vi "Navigation_Alex_auto.vi"() -> ()   [LabVIEW 2015]
uses:
  <vilib>/myRIO/Instrument Drivers/Utilities/Utilities.lvlib
  <vilib>/rvi/interface/nirviReadWriteControl/nirviReadWriteControl.xnode
  NiFpgaLv.dll
  <vilib>/Utility/error.llb/Error Cluster From Error Code.vi
  <vilib>/rvi/interface/Simulation/niFpgaSimulationCallBeginRW.vi
  <vilib>/rvi/errors/niLvFpgaAdjustHostInterfaceError.vi
  <vilib>/rvi/interface/nirviOpenFPGA/nirviOpenFPGA.xnode
  FPGA Bitfiles/NavigationProjec_FPGATarget2_FPGAMainNavigati_PWPHW8gwDxI.lvbitx
  <vilib>/FPGAPlugInAG/myRIO-1900/niLvFpga_Open_myRIO-1900.vi
  <vilib>/rvi/interface/common/dynamic/niFpgaDynamicAddResources.vi
  <vilib>/myRIO/Instrument Drivers/Onboard IO/PWM/typedefs/PWM Configuration.ctl
  <vilib>/myRIO/Instrument Drivers/Onboard IO/PWM/PWM.lvlib
  <vilib>/myRIO/Common/Instrument Driver Framework/myRIO v1.0/PWM/typedefs/PWM Channels Enum.ctl
  <vilib>/myRIO/Common/Instrument Driver Framework/Utilities/typedefs/Generic FPGA Reference.ctl
  <vilib>/myRIO/Common/Instrument Driver Framework/Utilities/typedefs/myRIO v1.0 Reference.ctl
  <vilib>/myRIO/Common/Instrument Driver Framework/Utilities/typedefs/Hardware Version Enum.ctl
  <vilib>/myRIO/Common/Instrument Driver Framework/Utilities/typedefs/myRIO Generic Hardware Reference.ctl
  <vilib>/myRIO/Instrument Drivers/Onboard IO/PWM/typedefs/PWM Reference.ctl
  <vilib>/myRIO/Instrument Drivers/Onboard IO/PWM/vis/myRIO PWM Open.xnode
  <vilib>/myRIO/Common/Instrument Driver Framework/myRIO v1.0/PWM/vis/myRIO v1.1 Open PWM.vi
  <vilib>/userdefined/High Color/nirio_resource_hc.ctl
panel:
  in  "Right PWM":dbl
  in  "Left PWM":dbl
  in  "Goal X":dbl
  out "Right Setpoint":dbl
  out "Current Angle":dbl
  out "Current Y":dbl
  out "Current X":dbl
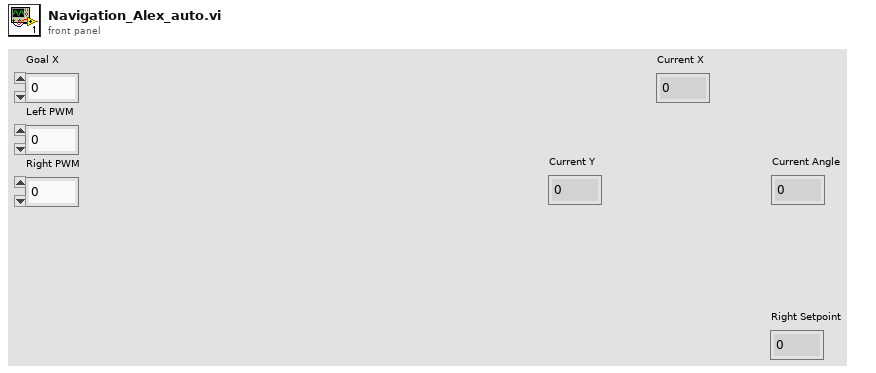
[diagram p1: front panel]
types:
  T1 = typedef "nirio_resource_hc.ctl" = tag
  T2 = typedef "Hardware Version Enum.ctl" = enum16{"Unknown", "myRIO-1900", "myRIO-1950", "roboRIO"}
  T3 = typedef "PWM.lvlib/PWM Reference.ctl" = cluster{"myRIO Reference":T4, "PWM Channels Enum":T7, "PWM Configuration":T8}
  T4 = typedef "myRIO Generic Hardware Reference.ctl" = cluster{"myRIO Model":T2, "myRIO Hardware Reference":T5}
  T5 = typedef "myRIO v1.0 Reference.ctl" = cluster{"Generic FPGA Reference":T6, "Allow multiple opens":bool}
  T6 = typedef "Generic FPGA Reference.ctl" = refnum<k20>
  T7 = typedef "PWM Channels Enum.ctl" = enum16{"Not Connected", "C/PWM0", "C/PWM1", "A/PWM0", "A/PWM1", "A/PWM2", "B/PWM0", "B/PWM1", "B/PWM2", "PWM/PWM0", "PWM/PWM1", "PWM/PWM2", "PWM/PWM3", "PWM/PWM4", "PWM/PWM5", "PWM/PWM6", "PWM/PWM7", "PWM/PWM8", "PWM/PWM9"}
  T8 = typedef "PWM.lvlib/PWM Configuration.ctl" = cluster{"Frequency":dbl, "Duty Cycle":dbl}
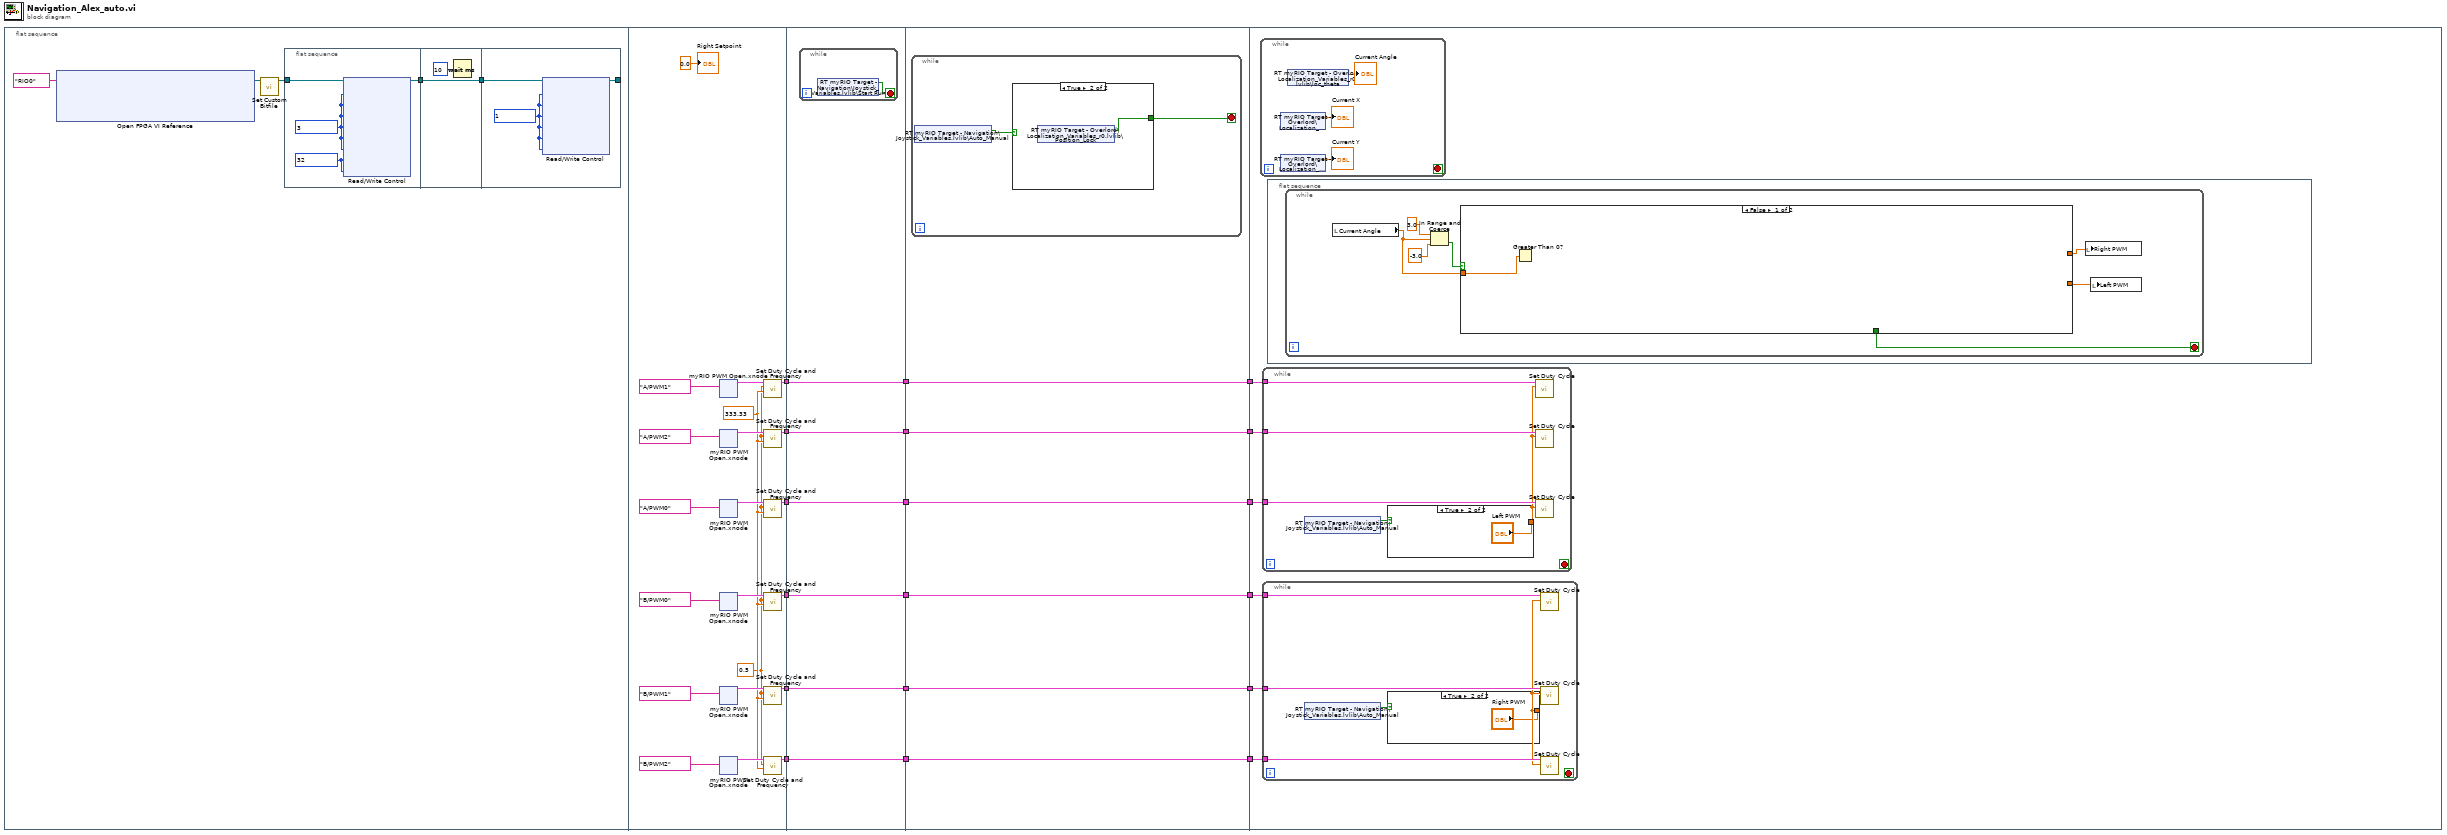
[diagram p0: block diagram]
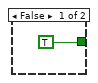
[diagram p2: hidden frame]
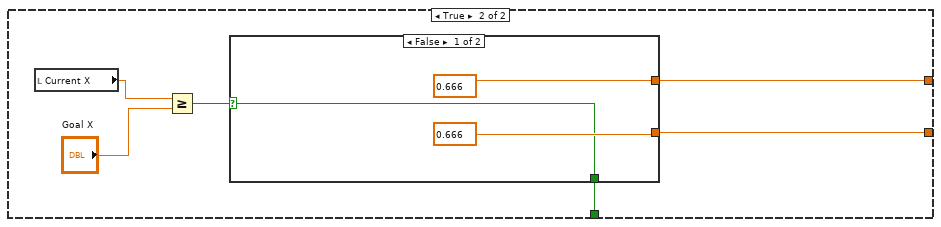
[diagram p3: hidden frame]
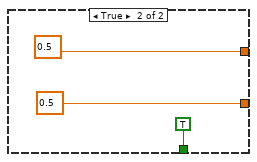
[diagram p4: hidden frame]
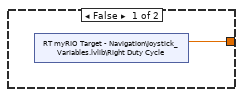
[diagram p5: hidden frame]
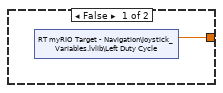
[diagram p6: hidden frame]
diagram:
  n1 = flat-sequence {
    tunnel: [w39] -> w18
    tunnel: [w38] -> w17
    tunnel: [w37] -> w16
    tunnel: [w36] -> w15
    tunnel: [w35] -> w14
    tunnel: [w34] -> w13
    tunnel: w18 -> [w155]
    tunnel: w17 -> [w154]
    tunnel: w16 -> [w153]
    tunnel: w15 -> [w152]
    tunnel: w14 -> [w151]
    tunnel: w13 -> [w150]
    tunnel: [w155] -> w12
    tunnel: [w154] -> w11
    tunnel: [w153] -> w10
    tunnel: [w152] -> w9
    tunnel: [w151] -> w8
    tunnel: [w150] -> w7
    tunnel: w12 -> [w162]
    tunnel: w11 -> [w161]
    tunnel: w10 -> [w160]
    tunnel: w9 -> [w159]
    tunnel: w8 -> [w158]
    tunnel: w7 -> [w157]
    tunnel: [w162] -> w6
    tunnel: [w161] -> w5
    tunnel: [w160] -> w4
    tunnel: [w159] -> w3
    tunnel: [w158] -> w2
    tunnel: [w157] -> w1
    tunnel: w1 -> [w169]
    tunnel: w2 -> [w168]
    tunnel: w3 -> [w167]
    tunnel: w4 -> [w170]
    tunnel: w5 -> [w171]
    tunnel: w6 -> [w172]
    frame #0 {
      n2 = xnode "Open FPGA VI Reference"("resource name"=tag "RIO0") -> ("FPGA VI Reference Out"=w20:refnum<k20>)  [unwired: 1 in, 1 out]
      n3 = call <vilib>:"Set Custom Bitfile.vi"("Custom FPGA Reference In"=w20) -> ("Custom FPGA Reference Out"=w21:refnum<k20>)  [unwired: 9 in, 1 out]
      n4 = flat-sequence {
        tunnel: w21 -> [w26]
        tunnel: [w24] -> w23
        tunnel: w23 -> [w28]
        tunnel: [w28] -> w22
        tunnel: w22 -> [w31]
        tunnel: [w30] -> _
        frame #0 {
          w25 = u8 32 ("SYS.SELECTA")
          w27 = u8 3 ("ENC.B_c.CNFG")
          n5 = xnode "Read/Write Control"("FPGA VI Reference In"=w26, "ENC.A_a.CNFG"=w27, "ENC.A_b.CNFG"=w27, "ENC.A_c.CNFG"=w27, "ENC.B_a.CNFG"=w27, "ENC.B_b.CNFG"=w27, "ENC.B_c.CNFG"=w27, "SYS.SELECTA"=w25, "SYS.SELECTB"=w25) -> ("FPGA VI Reference Out"=w24:refnum<k20>)  [unwired: 1 in, 1 out]
        }
        frame #1 {
          n6 = Wait (ms)(milliseconds to wait=u32 10) -> ()  [unwired: 1 out]
        }
        frame #2 {
          w32 = u8 1 ("ENC.B_c.CNFG")
          n7 = xnode "Read/Write Control"("FPGA VI Reference In"=w31, "ENC.A_a.CNFG"=w32, "ENC.A_b.CNFG"=w32, "ENC.A_c.CNFG"=w32, "ENC.B_a.CNFG"=w32, "ENC.B_b.CNFG"=w32, "ENC.B_c.CNFG"=w32) -> ("FPGA VI Reference Out"=w30:refnum<k20>)  [unwired: 1 in, 1 out]
        }
      }
    }
    frame #1 {
      w40 = 0.5
      w41 = 333.33
      n8 = xnode "myRIO PWM Open.xnode"("Channel Name"=tag "A/PWM1") -> ("PWM Ref Out"=w46:T3)  [unwired: 2 in, 1 out]
      n9 = xnode "myRIO PWM Open.xnode"("Channel Name"=tag "A/PWM2") -> ("PWM Ref Out"=w45:T3)  [unwired: 2 in, 1 out]
      n10 = xnode "myRIO PWM Open.xnode"("Channel Name"=tag "A/PWM0") -> ("PWM Ref Out"=w47:T3)  [unwired: 2 in, 1 out]
      n11 = xnode "myRIO PWM Open.xnode"("Channel Name"=tag "B/PWM0") -> ("PWM Ref Out"=w44:T3)  [unwired: 2 in, 1 out]
      n12 = xnode "myRIO PWM Open.xnode"("Channel Name"=tag "B/PWM1") -> ("PWM Ref Out"=w43:T3)  [unwired: 2 in, 1 out]
      n13 = xnode "myRIO PWM Open.xnode"("Channel Name"=tag "B/PWM2") -> ("PWM Ref Out"=w42:T3)  [unwired: 2 in, 1 out]
      n14 = call <vilib>:"Set Duty Cycle and Frequency.vi"("Frequency [Hz]"=w41, "Duty Cycle"=w40, "PWM Ref In"=w46) -> ("PWM Ref Out"=w38:T3)  [unwired: 6 in, 1 out]
      n15 = call <vilib>:"Set Duty Cycle and Frequency.vi"("Frequency [Hz]"=w41, "Duty Cycle"=w40, "PWM Ref In"=w45) -> ("PWM Ref Out"=w37:T3)  [unwired: 6 in, 1 out]
      n16 = call <vilib>:"Set Duty Cycle and Frequency.vi"("Frequency [Hz]"=w41, "Duty Cycle"=w40, "PWM Ref In"=w47) -> ("PWM Ref Out"=w39:T3)  [unwired: 6 in, 1 out]
      n17 = call <vilib>:"Set Duty Cycle and Frequency.vi"("Frequency [Hz]"=w41, "Duty Cycle"=w40, "PWM Ref In"=w44) -> ("PWM Ref Out"=w36:T3)  [unwired: 6 in, 1 out]
      n18 = call <vilib>:"Set Duty Cycle and Frequency.vi"("Frequency [Hz]"=w41, "Duty Cycle"=w40, "PWM Ref In"=w43) -> ("PWM Ref Out"=w35:T3)  [unwired: 6 in, 1 out]
      n19 = call <vilib>:"Set Duty Cycle and Frequency.vi"("Frequency [Hz]"=w41, "Duty Cycle"=w40, "PWM Ref In"=w42) -> ("PWM Ref Out"=w34:T3)  [unwired: 6 in, 1 out]
      "Right Setpoint" <- 0.0
    }
    frame #2 {
      n20 = while {
        stop <- w156 stop-if-true
        n21 = shared-variable "RT myRIO Target - Navigation\\Joystick_Variables.lvlib\\Start Run"() -> (w156:bool)  [unwired: 1 in, 1 out]
      }
    }
    frame #3 {
      n22 = while {
        stop <- w164 stop-if-true
        n23 = shared-variable "RT myRIO Target - Navigation\\Joystick_Variables.lvlib\\Auto_Manual"() -> (w163:bool)  [unwired: 1 in, 1 out]
        n24 = case shown="True" w163 {
          tunnel: [TRUE w166] -> w164
          frame False {
          }
          frame True {
            n25 = shared-variable "RT myRIO Target - Overlord\\Localization_Variables_r0.lvlib\\Position_Lock"() -> (w166:bool)  [unwired: 1 in, 1 out]
          }
        }
      }
    }
    frame #4 {
      n26 = while {
        stop <- _ stop-if-true
        n27 = shared-variable "RT myRIO Target - Overlord\\Localization_Variables_r0.lvlib\\loc_x"() -> (→"Current X":dbl)  [unwired: 1 in, 1 out]
        n28 = shared-variable "RT myRIO Target - Overlord\\Localization_Variables_r0.lvlib\\loc_y"() -> (→"Current Y":dbl)  [unwired: 1 in, 1 out]
        n29 = shared-variable "RT myRIO Target - Overlord\\Localization_Variables_r0.lvlib\\loc_theta"() -> (→"Current Angle":dbl)  [unwired: 1 in, 1 out]
      }
      n30 = while {
        tunnel: w172 -> [w204]
        tunnel: w171 -> [w203]
        tunnel: w170 -> [w202]
        stop <- _ stop-if-true
        n31 = shared-variable "RT myRIO Target - Navigation\\Joystick_Variables.lvlib\\Auto_Manual"() -> (w201:bool)  [unwired: 1 in, 1 out]
        n32 = case shown="True" w201 {
          tunnel: [w205 "Left PWM"] -> w200
          frame False {
            n33 = shared-variable "RT myRIO Target - Navigation\\Joystick_Variables.lvlib\\Left Duty Cycle"() -> (w205:dbl)  [unwired: 1 in, 1 out]
          }
          frame True {
          }
        }
        n34 = call <vilib>:"Set Duty Cycle.vi"("Duty Cycle"=w200, "PWM Ref In"=w203) -> ()  [unwired: 7 in, 2 out]
        n35 = call <vilib>:"Set Duty Cycle.vi"("Duty Cycle"=w200, "PWM Ref In"=w202) -> ()  [unwired: 7 in, 2 out]
        n36 = call <vilib>:"Set Duty Cycle.vi"("Duty Cycle"=w200, "PWM Ref In"=w204) -> ()  [unwired: 7 in, 2 out]
      }
      n37 = while {
        tunnel: w169 -> [w197]
        tunnel: w168 -> [w196]
        tunnel: w167 -> [w195]
        stop <- _ stop-if-true
        n38 = shared-variable "RT myRIO Target - Navigation\\Joystick_Variables.lvlib\\Auto_Manual"() -> (w194:bool)  [unwired: 1 in, 1 out]
        n39 = case shown="True" w194 {
          tunnel: [w198 "Right PWM"] -> w193
          frame False {
            n40 = shared-variable "RT myRIO Target - Navigation\\Joystick_Variables.lvlib\\Right Duty Cycle"() -> (w198:dbl)  [unwired: 1 in, 1 out]
          }
          frame True {
          }
        }
        n41 = call <vilib>:"Set Duty Cycle.vi"("Duty Cycle"=w193, "PWM Ref In"=w195) -> ()  [unwired: 7 in, 2 out]
        n42 = call <vilib>:"Set Duty Cycle.vi"("Duty Cycle"=w193, "PWM Ref In"=w196) -> ()  [unwired: 7 in, 2 out]
        n43 = call <vilib>:"Set Duty Cycle.vi"("Duty Cycle"=w193, "PWM Ref In"=w197) -> ()  [unwired: 7 in, 2 out]
      }
      n44 = flat-sequence {
        frame #0 {
          n45 = while {
            stop <- w174 stop-if-true
            n46 = local read "Current Angle"() -> (w173:dbl)
            n47 = In Range and Coerce(upper limit=3.0, x=w173, lower limit=-3.0) -> (In Range?=w177:bool)  [unwired: 1 out]
            n48 = case shown="False" w177 {
              tunnel: [_ w183] -> w176
              tunnel: [_ w182] -> w175
              tunnel: [_ w181] -> w174
              tunnel: w173 -> [w180 _]
              frame False {
                n49 = Greater Than 0?(x=w180) -> ()  [unwired: 1 out]
              }
              frame True {
                n50 = local read "Current X"() -> (w186:dbl)
                n51 = Greater Or Equal?(x=w186, y="Goal X") -> (x >= y?=w184:bool)
                n52 = case shown="False" w184 {
                  selector: w184 -> [w187 _]
                  tunnel: [0.666 0.5] -> w183
                  tunnel: [0.666 0.5] -> w182
                  tunnel: [w187 TRUE] -> w181
                  frame False {
                  }
                  frame True {
                  }
                }
              }
            }
            n53 = local write "Right PWM"(w176) -> ()
            n54 = local write "Left PWM"(w175) -> ()
          }
        }
      }
    }
  }
